vi "Lesson3 - While Loop timers.vi"() -> ()   [LabVIEW 2013]
panel:
  out "Numeric 2":i32
  out "Numeric":i32
  in  "Stop Button 2":bool
  in  "Stop Button":bool
  out "Waveform Chart 2":dbl(graph)
  out "Waveform Chart":dbl(graph)
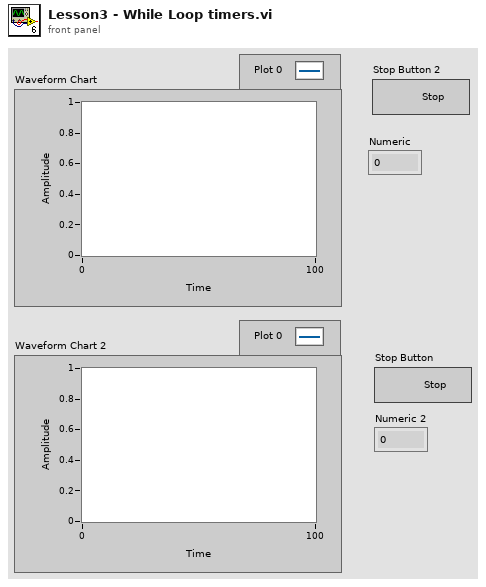
[diagram p1: front panel]
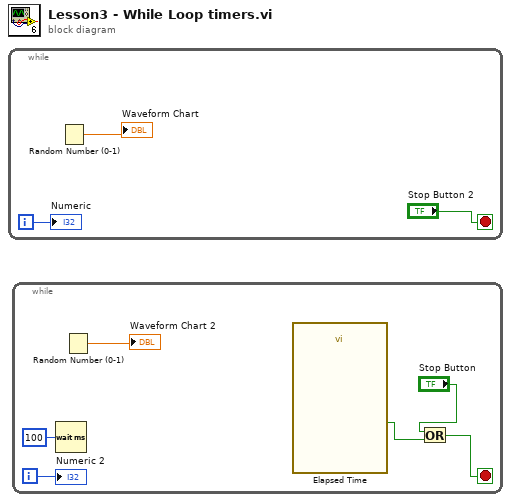
[diagram p0: block diagram]
diagram:
  n1 = while {
    i -> [w1]
    stop <- "Stop Button 2" stop-if-true
    n2 = Random Number (0-1)() -> (number: 0 to 1=→"Waveform Chart":dbl)
    "Numeric" <- w1
  }
  n3 = while {
    i -> [w4]
    stop <- w5 stop-if-true
    n4 = Wait (ms)(milliseconds to wait=u32 100) -> ()  [unwired: 1 out]
    n5 = Random Number (0-1)() -> (number: 0 to 1=→"Waveform Chart 2":dbl)
    n6 = call "Elapsed Time"() -> ("Time has Elapsed"=w8:bool)  [unwired: 12 in, 7 out]
    n7 = Or(x="Stop Button", y=w8) -> (x .or. y?=w5:bool)
    "Numeric 2" <- w4
  }
